vi "Configure Device.vi"(8 "error in (no error)":errorcluster, 10 "Max Beams":dbl, 11 "WS1040 in":refnum<class "WS1040.lvclass">) -> (0 "error out":errorcluster, 3 "WS1040 out":refnum<class "WS1040.lvclass">)   [LabVIEW 2020, in "WS1040.lvclass"]
doc: "Interface for configuring the device for testing"
uses:
  WS1040.lvclass
  Toggle 6.lvclass
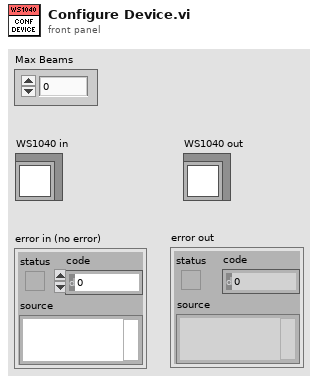
[diagram p1: front panel]
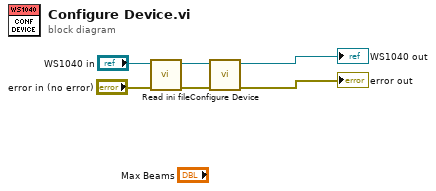
[diagram p0: block diagram]
diagram:
  n1 = call "Read ini file.vi"("Error In"="error in (no error)", "WS1040.lvclass"="WS1040 in") -> ("Error Out"=w1:errorcluster, "WS1040.lvclass Out"=w2:refnum<class "WS1040.lvclass">)  [unwired: 8 in]
  n2 = call-parent "Configure Device.vi"("error in (no error)"=w1, "Toggle 6 in"=w2) -> ("error out"=→"error out":errorcluster, "Toggle 6 out"=→"WS1040 out":refnum<class "WS1040.lvclass">)  [unwired: 8 in]
